vi "Eye Movement Analyser.vi"(7 "Data Output":T12) -> ()   [LabVIEW 2016] (continued)
                  w295 = T14[] [enum."Process Coils Data"] items=["--- System ---", "Panel Monitoring", "Check Save Status", "Initialize", "Initialise GUI", "Quit", "--- Import ---", "Desaccade Time Data", "Desaccade Time Data Background", "Paint Delete", "Load Batch Log File", "Make Batch List", "Update Batch List", "Delete Batch List", "Delete Temporary LVS", "Save Temporary LVS", "Check for Batch LVS", "Process 3D Chinchilla", "Find default parameter", "Mars3D old", "Chair", "EyeSeeCam", "Open last session", "Save RAW", "Auto Impulse Parameter", "Save Image", "Wireless", "Process Coils Data", "Process JHOC Data", "Process Animal Data", "Australian Data", "ASCII", "Mars 3D", "Mars 3D Training", "Position Mean Plugin", "plot generator plugin", "Human VOG system", "Optotrak", "spline", "COR", "galvanic", "Generate New Time Plot", "Make off and gains permanent", "Generate New Impulse Plot", "Defer Impulse Plot", "Fill Impulse Plot Data", "Scale Impulse Plot", "Un-Defer Impulse Plot", "Snap Impulse Cursor", "Extract Saccades", "Impulse Analyser", "NTA", "Acceleration", "Saccade Velocity", "Horizontal Align", "Vertical Align", "Delete Impulse", "Cut Before", "Cut After", "Filter Data", "Undo Last", "Redo", "Mean and STD", "Group Analyser", "Generate Report", "Phase Plots", "Gain and Phase", "Example Plugin", "Time Constant Plugin", "Export Data", "Export Time Series Data", "Append Data", "Save Data", "Load Data", "Cut in Range", "Keep in range", "Stop"] ("State Stack (out)")
                  n169 = event-data() -> ()  [unwired: 1 in, 7 out]
                }
                event "Impulse Analyser": Mouse Up {
                  w299 = T14[] [enum."Impulse Analyser", enum."Generate New Impulse Plot"] items=["--- System ---", "Panel Monitoring", "Check Save Status", "Initialize", "Initialise GUI", "Quit", "--- Import ---", "Desaccade Time Data", "Desaccade Time Data Background", "Paint Delete", "Load Batch Log File", "Make Batch List", "Update Batch List", "Delete Batch List", "Delete Temporary LVS", "Save Temporary LVS", "Check for Batch LVS", "Process 3D Chinchilla", "Find default parameter", "Mars3D old", "Chair", "EyeSeeCam", "Open last session", "Save RAW", "Auto Impulse Parameter", "Save Image", "Wireless", "Process Coils Data", "Process JHOC Data", "Process Animal Data", "Australian Data", "ASCII", "Mars 3D", "Mars 3D Training", "Position Mean Plugin", "plot generator plugin", "Human VOG system", "Optotrak", "spline", "COR", "galvanic", "Generate New Time Plot", "Make off and gains permanent", "Generate New Impulse Plot", "Defer Impulse Plot", "Fill Impulse Plot Data", "Scale Impulse Plot", "Un-Defer Impulse Plot", "Snap Impulse Cursor", "Extract Saccades", "Impulse Analyser", "NTA", "Acceleration", "Saccade Velocity", "Horizontal Align", "Vertical Align", "Delete Impulse", "Cut Before", "Cut After", "Filter Data", "Undo Last", "Redo", "Mean and STD", "Group Analyser", "Generate Report", "Phase Plots", "Gain and Phase", "Example Plugin", "Time Constant Plugin", "Export Data", "Export Time Series Data", "Append Data", "Save Data", "Load Data", "Cut in Range", "Keep in range", "Stop"] ("State Stack (out)")
                  n170 = event-data() -> ()  [unwired: 1 in, 7 out]
                  n171 = local write "Trace"(0 ("Trace")) -> ()
                }
                event "Generate New Plot": Mouse Up {
                  w302 = T14[] [enum."Generate New Time Plot"] items=["--- System ---", "Panel Monitoring", "Check Save Status", "Initialize", "Initialise GUI", "Quit", "--- Import ---", "Desaccade Time Data", "Desaccade Time Data Background", "Paint Delete", "Load Batch Log File", "Make Batch List", "Update Batch List", "Delete Batch List", "Delete Temporary LVS", "Save Temporary LVS", "Check for Batch LVS", "Process 3D Chinchilla", "Find default parameter", "Mars3D old", "Chair", "EyeSeeCam", "Open last session", "Save RAW", "Auto Impulse Parameter", "Save Image", "Wireless", "Process Coils Data", "Process JHOC Data", "Process Animal Data", "Australian Data", "ASCII", "Mars 3D", "Mars 3D Training", "Position Mean Plugin", "plot generator plugin", "Human VOG system", "Optotrak", "spline", "COR", "galvanic", "Generate New Time Plot", "Make off and gains permanent", "Generate New Impulse Plot", "Defer Impulse Plot", "Fill Impulse Plot Data", "Scale Impulse Plot", "Un-Defer Impulse Plot", "Snap Impulse Cursor", "Extract Saccades", "Impulse Analyser", "NTA", "Acceleration", "Saccade Velocity", "Horizontal Align", "Vertical Align", "Delete Impulse", "Cut Before", "Cut After", "Filter Data", "Undo Last", "Redo", "Mean and STD", "Group Analyser", "Generate Report", "Phase Plots", "Gain and Phase", "Example Plugin", "Time Constant Plugin", "Export Data", "Export Time Series Data", "Append Data", "Save Data", "Load Data", "Cut in Range", "Keep in range", "Stop"] ("State Stack (out)")
                  n172 = event-data() -> ()  [unwired: 1 in, 7 out]
                }
                event "Impulse Plane": Value Change {
                  n173 = event-data() -> ("NewVal"=w305:bool)  [unwired: 1 in, 4 out]
                  n174 = Select(t=T16."Enabled" ("Disabled"), s=w305, f=T16."Disabled and Grayed Out" ("Disabled")) -> (s? t:f=w309:T16)
                  n175 = property on="Trigger Channel (Other)" class="Ring (strict)"("DisabledEnum"=w309, "Visible"=TRUE) -> ()  [unwired: 2 in, 2 out]
                  n176 = local write "Other Trigger channel"(w305) -> ()
                  n177 = case shown="False" w305 {
                    frame False {
                      n178 = local write "Impulse Plane 2"(T9."Yaw" ("Impulse Plane")) -> ()
                    }
                    frame True {
                      n179 = local write "Impulse Plane 2"(T9."Other" ("Impulse Plane")) -> ()
                    }
                  }
                  n180 = local write "Trace"(0 ("Trace")) -> ()
                }
                event "Trace": Value Change {
                  w316 = T14[] [enum."Generate New Impulse Plot"] items=["--- System ---", "Panel Monitoring", "Check Save Status", "Initialize", "Initialise GUI", "Quit", "--- Import ---", "Desaccade Time Data", "Desaccade Time Data Background", "Paint Delete", "Load Batch Log File", "Make Batch List", "Update Batch List", "Delete Batch List", "Delete Temporary LVS", "Save Temporary LVS", "Check for Batch LVS", "Process 3D Chinchilla", "Find default parameter", "Mars3D old", "Chair", "EyeSeeCam", "Open last session", "Save RAW", "Auto Impulse Parameter", "Save Image", "Wireless", "Process Coils Data", "Process JHOC Data", "Process Animal Data", "Australian Data", "ASCII", "Mars 3D", "Mars 3D Training", "Position Mean Plugin", "plot generator plugin", "Human VOG system", "Optotrak", "spline", "COR", "galvanic", "Generate New Time Plot", "Make off and gains permanent", "Generate New Impulse Plot", "Defer Impulse Plot", "Fill Impulse Plot Data", "Scale Impulse Plot", "Un-Defer Impulse Plot", "Snap Impulse Cursor", "Extract Saccades", "Impulse Analyser", "NTA", "Acceleration", "Saccade Velocity", "Horizontal Align", "Vertical Align", "Delete Impulse", "Cut Before", "Cut After", "Filter Data", "Undo Last", "Redo", "Mean and STD", "Group Analyser", "Generate Report", "Phase Plots", "Gain and Phase", "Example Plugin", "Time Constant Plugin", "Export Data", "Export Time Series Data", "Append Data", "Save Data", "Load Data", "Cut in Range", "Keep in range", "Stop"] ("State Stack (out)")
                  n181 = event-data() -> ()  [unwired: 1 in, 5 out]
                }
                event "Analyze Saccades": Mouse Down {
                  w319 = T14[] [enum."Desaccade Time Data"] items=["--- System ---", "Panel Monitoring", "Check Save Status", "Initialize", "Initialise GUI", "Quit", "--- Import ---", "Desaccade Time Data", "Desaccade Time Data Background", "Paint Delete", "Load Batch Log File", "Make Batch List", "Update Batch List", "Delete Batch List", "Delete Temporary LVS", "Save Temporary LVS", "Check for Batch LVS", "Process 3D Chinchilla", "Find default parameter", "Mars3D old", "Chair", "EyeSeeCam", "Open last session", "Save RAW", "Auto Impulse Parameter", "Save Image", "Wireless", "Process Coils Data", "Process JHOC Data", "Process Animal Data", "Australian Data", "ASCII", "Mars 3D", "Mars 3D Training", "Position Mean Plugin", "plot generator plugin", "Human VOG system", "Optotrak", "spline", "COR", "galvanic", "Generate New Time Plot", "Make off and gains permanent", "Generate New Impulse Plot", "Defer Impulse Plot", "Fill Impulse Plot Data", "Scale Impulse Plot", "Un-Defer Impulse Plot", "Snap Impulse Cursor", "Extract Saccades", "Impulse Analyser", "NTA", "Acceleration", "Saccade Velocity", "Horizontal Align", "Vertical Align", "Delete Impulse", "Cut Before", "Cut After", "Filter Data", "Undo Last", "Redo", "Mean and STD", "Group Analyser", "Generate Report", "Phase Plots", "Gain and Phase", "Example Plugin", "Time Constant Plugin", "Export Data", "Export Time Series Data", "Append Data", "Save Data", "Load Data", "Cut in Range", "Keep in range", "Stop"] ("State Stack (out)")
                  n182 = event-data() -> ()  [unwired: 1 in, 7 out]
                }
                event "Capture Saccade": Value Change {
                  w321 = T14[] [enum."Generate New Impulse Plot"] items=["--- System ---", "Panel Monitoring", "Check Save Status", "Initialize", "Initialise GUI", "Quit", "--- Import ---", "Desaccade Time Data", "Desaccade Time Data Background", "Paint Delete", "Load Batch Log File", "Make Batch List", "Update Batch List", "Delete Batch List", "Delete Temporary LVS", "Save Temporary LVS", "Check for Batch LVS", "Process 3D Chinchilla", "Find default parameter", "Mars3D old", "Chair", "EyeSeeCam", "Open last session", "Save RAW", "Auto Impulse Parameter", "Save Image", "Wireless", "Process Coils Data", "Process JHOC Data", "Process Animal Data", "Australian Data", "ASCII", "Mars 3D", "Mars 3D Training", "Position Mean Plugin", "plot generator plugin", "Human VOG system", "Optotrak", "spline", "COR", "galvanic", "Generate New Time Plot", "Make off and gains permanent", "Generate New Impulse Plot", "Defer Impulse Plot", "Fill Impulse Plot Data", "Scale Impulse Plot", "Un-Defer Impulse Plot", "Snap Impulse Cursor", "Extract Saccades", "Impulse Analyser", "NTA", "Acceleration", "Saccade Velocity", "Horizontal Align", "Vertical Align", "Delete Impulse", "Cut Before", "Cut After", "Filter Data", "Undo Last", "Redo", "Mean and STD", "Group Analyser", "Generate Report", "Phase Plots", "Gain and Phase", "Example Plugin", "Time Constant Plugin", "Export Data", "Export Time Series Data", "Append Data", "Save Data", "Load Data", "Cut in Range", "Keep in range", "Stop"] ("State Stack (out)")
                  n183 = event-data() -> ()  [unwired: 1 in, 5 out]
                }
                event "Options", "Help": Value Change {
                  n184 = event-data() -> ()  [unwired: 1 in, 5 out]
                  n185 = local read "Options"() -> (w326:bool)
                  n186 = case shown="False" w326 {
                    tunnel: [w327 enum32{"Page 1", "Page 3", "Page 2"}."Page 2" ("Tab Control Impuls")] -> w325
                    frame False {
                      n187 = local read "Help"() -> (w328:bool)
                      n188 = case shown="True" w328 {
                        tunnel: [enum32{"Page 1", "Page 3", "Page 2"}."Page 1" ("Tab Control Impuls") enum32{"Page 1", "Page 3", "Page 2"}."Page 3" ("Tab Control Impuls")] -> w327
                        frame False {
                        }
                        frame True {
                        }
                      }
                    }
                    frame True {
                    }
                  }
                  n189 = local write "Tab Control Impuls"(w325) -> ()
                }
                event "Impulse Characteristic from Cursor": Mouse Up {
                  n190 = event-data() -> ()  [unwired: 1 in, 7 out]
                  n191 = property on="Time series Trace" class="WFGraph (strict)"("Active Cursor"=u32 1) -> ("Cursor.Cursor X"=w338:dbl, "Cursor.Cursor Y"=w345:dbl)  [unwired: 2 in, 2 out]
                  n192 = property on="Time series Trace" class="WFGraph (strict)"("Active Cursor"=u32 0) -> ("Cursor.Cursor X"=w335:dbl, "Cursor.Cursor Y"=w346:dbl)  [unwired: 2 in, 2 out]
                  n193 = Multiply(x=w338, y=1000.0) -> (x*y=w337:dbl)
                  n194 = Multiply(x=w335, y=1000.0) -> (x*y=w334:dbl)
                  n195 = property on="Impulse surround" class="Clust (strict)"() -> ("Value"=w353:T6)  [unwired: 2 in, 2 out]
                  n196 = Subtract(x=w337, y=w334) -> (x-y=w350:dbl)
                  n197 = Max & Min(x=w346, y=w345) -> (max(x,y)=w343:dbl)  [unwired: 1 out]
                  n198 = Divide(x=w350, y=2.0) -> (x/y=w358:dbl)
                  n199 = Multiply(x=w350, y=0.2) -> (x*y=w347:dbl)
                  n200 = Multiply(x=w350, y=1.2) -> (x*y=w348:dbl)
                  n201 = property on="Impulse Characteristics" class="Clust (strict)"() -> ("Value"=w355:T7)  [unwired: 2 in, 2 out]
                  n202 = Bundle By Name(cluster=w353, "Pre Impulse (ms)"=w347, "Post Impulse (ms)"=w348) -> (w352:T6)
                  n203 = Multiply(x=w343, y=0.7) -> (x*y=w341:dbl)
                  n204 = Multiply(x=w343, y=1.3) -> (x*y=w340:dbl)
                  n205 = Multiply(x=w358, y=0.8) -> (x*y=w354:dbl)
                  n206 = property on="Impulse surround" class="Clust (strict)"("Value"=w352) -> ()  [unwired: 2 in, 2 out]
                  n207 = Bundle By Name(cluster=w355, "Min Vel /Trigger"=w341, "Maximum Velocity"=w340, "Width / Offset (ms)"=w354) -> (w356:T7)
                  n208 = property on="Impulse Characteristics" class="Clust (strict)"("Value"=w356) -> ()  [unwired: 2 in, 2 out]
                }
                event "Add Autosort": Mouse Up {
                  n209 = event-data() -> ()  [unwired: 1 in, 7 out]
                  n210 = property on="Autosize Parameter Set" class="Ring (strict)"() -> ("Value"=w365:i8)  [unwired: 2 in, 2 out]
                  n211 = Equal To 0?(x=w365) -> (x = 0?=w364:bool)
                  n212 = case shown="False" w364 {
                    frame False {
                      w366 = TRUE ("Visible")
                      w367 = FALSE ("Visible")
                      w369 = TRUE ("Visible")
                      n213 = property on="Add Autosort OK" class="Bool (strict)"("Visible"=w369) -> ()  [unwired: 2 in, 2 out]
                      n214 = property on="Add Autosort Cancel" class="Bool (strict)"("Visible"=w369) -> ()  [unwired: 2 in, 2 out]
                      n215 = property on="Add Autosort" class="Bool (strict)"("Visible"=w367) -> ()  [unwired: 2 in, 2 out]
                      n216 = property on="Del Autosort" class="Bool (strict)"("Visible"=w367) -> ()  [unwired: 2 in, 2 out]
                      n217 = property on="Autosort Name" class="Str"("Visible"=w369, "Value"="" ("Autosort Name")) -> ()  [unwired: 2 in, 2 out]
                      n218 = property on="Default" class="Bool (strict)"("Visible"=w366, "Value"=w366) -> ()  [unwired: 2 in, 2 out]
                    }
                    frame True {
                      n219 = One Button Dialog(message="No Parameter-Set selected! Please select an Auto-Sort Parameter-Set by using a Load-Data Program like Mars 3D. ") -> ()  [unwired: 1 in, 1 out]
                    }
                  }
                }
                event "Add Autosort Cancel": Mouse Up {
                  w372 = FALSE ("Visible")
                  w374 = TRUE ("Visible")
                  w375 = FALSE ("Visible")
                  n220 = event-data() -> ()  [unwired: 1 in, 7 out]
                  n221 = property on="Add Autosort OK" class="Bool (strict)"("Visible"=w375) -> ()  [unwired: 2 in, 2 out]
                  n222 = property on="Add Autosort Cancel" class="Bool (strict)"("Visible"=w375) -> ()  [unwired: 2 in, 2 out]
                  n223 = property on="Add Autosort" class="Bool (strict)"("Visible"=w374) -> ()  [unwired: 2 in, 2 out]
                  n224 = property on="Autosort Name" class="Str"("Visible"=w375) -> ()  [unwired: 2 in, 2 out]
                  n225 = property on="Del Autosort" class="Bool (strict)"("Visible"=w374) -> ()  [unwired: 2 in, 2 out]
                  n226 = property on="Default" class="Bool (strict)"("Visible"=w372, "Value"=w372) -> ()  [unwired: 2 in, 2 out]
                }
                event "Add Autosort OK": Mouse Up {
                  w387 = TRUE ("Visible")
                  w388 = FALSE ("Visible")
                  n227 = event-data() -> ()  [unwired: 1 in, 7 out]
                  n228 = control-ref of="Autosize Parameter Set"() -> (w383:refnum<vi>)
                  n229 = control-ref of="Autosort Name"() -> (w381:refnum<vi>)
                  n230 = control-ref of="Cross Correlation"() -> (w376:refnum<vi>)
                  n231 = control-ref of="Impulse surround"() -> (w380:refnum<vi>)
                  n232 = control-ref of="Impulse Characteristics"() -> (w379:refnum<vi>)
                  n233 = control-ref of="Trigger Channel (Other)"() -> (w378:refnum<vi>)
                  n234 = control-ref of="Impulse Plane"() -> (w377:refnum<vi>)
                  n235 = call "Add Autosort OK pressed.vi"("Ring in"=w383, "Default"="Default", "Data OUT"=w386, "Str Refnum"=w381, "reference 5"=w376, "reference"=w380, "reference 2"=w379, "reference 3"=w378, "reference 4"=w377) -> ()  [unwired: 7 in]
                  n236 = property on="Autosort Name" class="Str"("Visible"=w388) -> ()  [unwired: 2 in, 2 out]
                  n237 = property on="Add Autosort OK" class="Bool (strict)"("Visible"=w388) -> ()  [unwired: 2 in, 2 out]
                  n238 = property on="Add Autosort Cancel" class="Bool (strict)"("Visible"=w388) -> ()  [unwired: 2 in, 2 out]
                  n239 = property on="Add Autosort" class="Bool (strict)"("Visible"=w387) -> ()  [unwired: 2 in, 2 out]
                  n240 = property on="Del Autosort" class="Bool (strict)"("Visible"=w387) -> ()  [unwired: 2 in, 2 out]
                  n241 = property on="Default" class="Bool (strict)"("Visible"=FALSE) -> ()  [unwired: 2 in, 2 out]
                }
                event "Del Autosort": Mouse Up {
                  w393 = TRUE ("Visible")
                  w394 = FALSE ("Visible")
                  n242 = event-data() -> ()  [unwired: 1 in, 7 out]
                  n243 = control-ref of="Autosize Parameter Set"() -> (w390:refnum<vi>)
                  n244 = control-ref of="Auto Sort Parameter"() -> (w389:refnum<vi>)
                  n245 = call "Autosort Delete pressed.vi"("Data OUT"=w392, "reference"=w389, "Ring in"=w390) -> ()  [unwired: 9 in]
                  n246 = property on="Autosort Name" class="Str"("Visible"=w394) -> ()  [unwired: 2 in, 2 out]
                  n247 = property on="Add Autosort OK" class="Bool (strict)"("Visible"=w394) -> ()  [unwired: 2 in, 2 out]
                  n248 = property on="Add Autosort Cancel" class="Bool (strict)"("Visible"=w394) -> ()  [unwired: 2 in, 2 out]
                  n249 = property on="Add Autosort" class="Bool (strict)"("Visible"=w393) -> ()  [unwired: 2 in, 2 out]
                  n250 = property on="Del Autosort" class="Bool (strict)"("Visible"=w393) -> ()  [unwired: 2 in, 2 out]
                }
                event "Autosize Parameter Set": Value Change {
                  n251 = event-data() -> ("NewVal"=w401:i8)  [unwired: 1 in, 4 out]
                  n252 = Not Equal?(x=w401, y=i8 0) -> (x != y?=w395:bool)
                  n253 = property on="Add Autosort" class="Bool (strict)"("Visible"=w395) -> ()  [unwired: 2 in, 2 out]
                  n254 = property on="Del Autosort" class="Bool (strict)"("Visible"=w395) -> ()  [unwired: 2 in, 2 out]
                  n255 = control-ref of="Auto Sort Parameter"() -> (w396:refnum<vi>)
                  n256 = call "Autosort Parameter Set selected.vi"("NewVal"=w401, "Data OUT"=w399, "Ring in"=w396) -> ("State stack IN"=w398:T14[])  [unwired: 8 in]
                }
                event "Filter Data": Mouse Up {
                  w403 = T14[] [enum."Filter Data", enum."Generate New Time Plot"] items=["--- System ---", "Panel Monitoring", "Check Save Status", "Initialize", "Initialise GUI", "Quit", "--- Import ---", "Desaccade Time Data", "Desaccade Time Data Background", "Paint Delete", "Load Batch Log File", "Make Batch List", "Update Batch List", "Delete Batch List", "Delete Temporary LVS", "Save Temporary LVS", "Check for Batch LVS", "Process 3D Chinchilla", "Find default parameter", "Mars3D old", "Chair", "EyeSeeCam", "Open last session", "Save RAW", "Auto Impulse Parameter", "Save Image", "Wireless", "Process Coils Data", "Process JHOC Data", "Process Animal Data", "Australian Data", "ASCII", "Mars 3D", "Mars 3D Training", "Position Mean Plugin", "plot generator plugin", "Human VOG system", "Optotrak", "spline", "COR", "galvanic", "Generate New Time Plot", "Make off and gains permanent", "Generate New Impulse Plot", "Defer Impulse Plot", "Fill Impulse Plot Data", "Scale Impulse Plot", "Un-Defer Impulse Plot", "Snap Impulse Cursor", "Extract Saccades", "Impulse Analyser", "NTA", "Acceleration", "Saccade Velocity", "Horizontal Align", "Vertical Align", "Delete Impulse", "Cut Before", "Cut After", "Filter Data", "Undo Last", "Redo", "Mean and STD", "Group Analyser", "Generate Report", "Phase Plots", "Gain and Phase", "Example Plugin", "Time Constant Plugin", "Export Data", "Export Time Series Data", "Append Data", "Save Data", "Load Data", "Cut in Range", "Keep in range", "Stop"] ("State Stack (out)")
                  n257 = event-data() -> ()  [unwired: 1 in, 7 out]
                }
                event "Generate New Impulse Plot": Mouse Up {
                  w406 = T14[] [enum."Generate New Impulse Plot"] items=["--- System ---", "Panel Monitoring", "Check Save Status", "Initialize", "Initialise GUI", "Quit", "--- Import ---", "Desaccade Time Data", "Desaccade Time Data Background", "Paint Delete", "Load Batch Log File", "Make Batch List", "Update Batch List", "Delete Batch List", "Delete Temporary LVS", "Save Temporary LVS", "Check for Batch LVS", "Process 3D Chinchilla", "Find default parameter", "Mars3D old", "Chair", "EyeSeeCam", "Open last session", "Save RAW", "Auto Impulse Parameter", "Save Image", "Wireless", "Process Coils Data", "Process JHOC Data", "Process Animal Data", "Australian Data", "ASCII", "Mars 3D", "Mars 3D Training", "Position Mean Plugin", "plot generator plugin", "Human VOG system", "Optotrak", "spline", "COR", "galvanic", "Generate New Time Plot", "Make off and gains permanent", "Generate New Impulse Plot", "Defer Impulse Plot", "Fill Impulse Plot Data", "Scale Impulse Plot", "Un-Defer Impulse Plot", "Snap Impulse Cursor", "Extract Saccades", "Impulse Analyser", "NTA", "Acceleration", "Saccade Velocity", "Horizontal Align", "Vertical Align", "Delete Impulse", "Cut Before", "Cut After", "Filter Data", "Undo Last", "Redo", "Mean and STD", "Group Analyser", "Generate Report", "Phase Plots", "Gain and Phase", "Example Plugin", "Time Constant Plugin", "Export Data", "Export Time Series Data", "Append Data", "Save Data", "Load Data", "Cut in Range", "Keep in range", "Stop"] ("State Stack (out)")
                  n258 = event-data() -> ()  [unwired: 1 in, 7 out]
                }
                event "Horizontal Align": Mouse Up {
                  w409 = T14[] [enum."Horizontal Align", enum."Generate New Impulse Plot"] items=["--- System ---", "Panel Monitoring", "Check Save Status", "Initialize", "Initialise GUI", "Quit", "--- Import ---", "Desaccade Time Data", "Desaccade Time Data Background", "Paint Delete", "Load Batch Log File", "Make Batch List", "Update Batch List", "Delete Batch List", "Delete Temporary LVS", "Save Temporary LVS", "Check for Batch LVS", "Process 3D Chinchilla", "Find default parameter", "Mars3D old", "Chair", "EyeSeeCam", "Open last session", "Save RAW", "Auto Impulse Parameter", "Save Image", "Wireless", "Process Coils Data", "Process JHOC Data", "Process Animal Data", "Australian Data", "ASCII", "Mars 3D", "Mars 3D Training", "Position Mean Plugin", "plot generator plugin", "Human VOG system", "Optotrak", "spline", "COR", "galvanic", "Generate New Time Plot", "Make off and gains permanent", "Generate New Impulse Plot", "Defer Impulse Plot", "Fill Impulse Plot Data", "Scale Impulse Plot", "Un-Defer Impulse Plot", "Snap Impulse Cursor", "Extract Saccades", "Impulse Analyser", "NTA", "Acceleration", "Saccade Velocity", "Horizontal Align", "Vertical Align", "Delete Impulse", "Cut Before", "Cut After", "Filter Data", "Undo Last", "Redo", "Mean and STD", "Group Analyser", "Generate Report", "Phase Plots", "Gain and Phase", "Example Plugin", "Time Constant Plugin", "Export Data", "Export Time Series Data", "Append Data", "Save Data", "Load Data", "Cut in Range", "Keep in range", "Stop"] ("State Stack (out)")
                  n259 = event-data() -> ()  [unwired: 1 in, 7 out]
                }
                event "Vertical Align": Mouse Up {
                  w412 = T14[] [enum."Vertical Align", enum."Generate New Impulse Plot"] items=["--- System ---", "Panel Monitoring", "Check Save Status", "Initialize", "Initialise GUI", "Quit", "--- Import ---", "Desaccade Time Data", "Desaccade Time Data Background", "Paint Delete", "Load Batch Log File", "Make Batch List", "Update Batch List", "Delete Batch List", "Delete Temporary LVS", "Save Temporary LVS", "Check for Batch LVS", "Process 3D Chinchilla", "Find default parameter", "Mars3D old", "Chair", "EyeSeeCam", "Open last session", "Save RAW", "Auto Impulse Parameter", "Save Image", "Wireless", "Process Coils Data", "Process JHOC Data", "Process Animal Data", "Australian Data", "ASCII", "Mars 3D", "Mars 3D Training", "Position Mean Plugin", "plot generator plugin", "Human VOG system", "Optotrak", "spline", "COR", "galvanic", "Generate New Time Plot", "Make off and gains permanent", "Generate New Impulse Plot", "Defer Impulse Plot", "Fill Impulse Plot Data", "Scale Impulse Plot", "Un-Defer Impulse Plot", "Snap Impulse Cursor", "Extract Saccades", "Impulse Analyser", "NTA", "Acceleration", "Saccade Velocity", "Horizontal Align", "Vertical Align", "Delete Impulse", "Cut Before", "Cut After", "Filter Data", "Undo Last", "Redo", "Mean and STD", "Group Analyser", "Generate Report", "Phase Plots", "Gain and Phase", "Example Plugin", "Time Constant Plugin", "Export Data", "Export Time Series Data", "Append Data", "Save Data", "Load Data", "Cut in Range", "Keep in range", "Stop"] ("State Stack (out)")
                  n260 = event-data() -> ()  [unwired: 1 in, 7 out]
                }
                event "Delete Impulse": Mouse Up {
                  w415 = T14[] [enum."Delete Impulse", enum."Generate New Impulse Plot"] items=["--- System ---", "Panel Monitoring", "Check Save Status", "Initialize", "Initialise GUI", "Quit", "--- Import ---", "Desaccade Time Data", "Desaccade Time Data Background", "Paint Delete", "Load Batch Log File", "Make Batch List", "Update Batch List", "Delete Batch List", "Delete Temporary LVS", "Save Temporary LVS", "Check for Batch LVS", "Process 3D Chinchilla", "Find default parameter", "Mars3D old", "Chair", "EyeSeeCam", "Open last session", "Save RAW", "Auto Impulse Parameter", "Save Image", "Wireless", "Process Coils Data", "Process JHOC Data", "Process Animal Data", "Australian Data", "ASCII", "Mars 3D", "Mars 3D Training", "Position Mean Plugin", "plot generator plugin", "Human VOG system", "Optotrak", "spline", "COR", "galvanic", "Generate New Time Plot", "Make off and gains permanent", "Generate New Impulse Plot", "Defer Impulse Plot", "Fill Impulse Plot Data", "Scale Impulse Plot", "Un-Defer Impulse Plot", "Snap Impulse Cursor", "Extract Saccades", "Impulse Analyser", "NTA", "Acceleration", "Saccade Velocity", "Horizontal Align", "Vertical Align", "Delete Impulse", "Cut Before", "Cut After", "Filter Data", "Undo Last", "Redo", "Mean and STD", "Group Analyser", "Generate Report", "Phase Plots", "Gain and Phase", "Example Plugin", "Time Constant Plugin", "Export Data", "Export Time Series Data", "Append Data", "Save Data", "Load Data", "Cut in Range", "Keep in range", "Stop"] ("State Stack (out)")
                  n261 = event-data() -> ()  [unwired: 1 in, 7 out]
                }
                event Key Down {
                  n262 = event-data() -> ("Char"=w422:i16, "VKey"=w426:T33, "PlatMods"=w417:T34)  [unwired: 1 in, 6 out]
                  n263 = Type Cast(type="", x=w422) -> (*(type *) &x=w420:string)
                  n264 = String Subset(string=w420, offset (0)=1) -> (substring=w418:string)  [unwired: 1 in]
                  n265 = case shown="\"Delete\", \"Escape\"" w426 {
                    tunnel: [w429 w435 w441 w443 _] -> w424
                    tunnel: w418 -> [w428 _ _ _ _]
                    tunnel: w417 -> [w427 _ _ _ _]
                    frame "ASCII", Default {
                      n266 = case shown="\"g\"" w428 {
                        tunnel: [w430 w433] -> w429
                        tunnel: w427 -> [_ w432]
                        frame "", Default {
                          w430 = T14[] [enum."Panel Monitoring"] items=["--- System ---", "Panel Monitoring", "Check Save Status", "Initialize", "Initialise GUI", "Quit", "--- Import ---", "Desaccade Time Data", "Desaccade Time Data Background", "Paint Delete", "Load Batch Log File", "Make Batch List", "Update Batch List", "Delete Batch List", "Delete Temporary LVS", "Save Temporary LVS", "Check for Batch LVS", "Process 3D Chinchilla", "Find default parameter", "Mars3D old", "Chair", "EyeSeeCam", "Open last session", "Save RAW", "Auto Impulse Parameter", "Save Image", "Wireless", "Process Coils Data", "Process JHOC Data", "Process Animal Data", "Australian Data", "ASCII", "Mars 3D", "Mars 3D Training", "Position Mean Plugin", "plot generator plugin", "Human VOG system", "Optotrak", "spline", "COR", "galvanic", "Generate New Time Plot", "Make off and gains permanent", "Generate New Impulse Plot", "Defer Impulse Plot", "Fill Impulse Plot Data", "Scale Impulse Plot", "Un-Defer Impulse Plot", "Snap Impulse Cursor", "Extract Saccades", "Impulse Analyser", "NTA", "Acceleration", "Saccade Velocity", "Horizontal Align", "Vertical Align", "Delete Impulse", "Cut Before", "Cut After", "Filter Data", "Undo Last", "Redo", "Mean and STD", "Group Analyser", "Generate Report", "Phase Plots", "Gain and Phase", "Example Plugin", "Time Constant Plugin", "Export Data", "Export Time Series Data", "Append Data", "Save Data", "Load Data", "Cut in Range", "Keep in range", "Stop"] ("State Stack (out)")
                        }
                        frame "g" {
                          n267 = Unbundle By Name(w432) -> ("Ctrl"=w431:bool)
                          n268 = case shown="True" w431 {
                            tunnel: [_ w434] -> w433
                            frame False {
                            }
                            frame True {
                              w434 = T14[] [enum."Gain and Phase"] items=["--- System ---", "Panel Monitoring", "Check Save Status", "Initialize", "Initialise GUI", "Quit", "--- Import ---", "Desaccade Time Data", "Desaccade Time Data Background", "Paint Delete", "Load Batch Log File", "Make Batch List", "Update Batch List", "Delete Batch List", "Delete Temporary LVS", "Save Temporary LVS", "Check for Batch LVS", "Process 3D Chinchilla", "Find default parameter", "Mars3D old", "Chair", "EyeSeeCam", "Open last session", "Save RAW", "Auto Impulse Parameter", "Save Image", "Wireless", "Process Coils Data", "Process JHOC Data", "Process Animal Data", "Australian Data", "ASCII", "Mars 3D", "Mars 3D Training", "Position Mean Plugin", "plot generator plugin", "Human VOG system", "Optotrak", "spline", "COR", "galvanic", "Generate New Time Plot", "Make off and gains permanent", "Generate New Impulse Plot", "Defer Impulse Plot", "Fill Impulse Plot Data", "Scale Impulse Plot", "Un-Defer Impulse Plot", "Snap Impulse Cursor", "Extract Saccades", "Impulse Analyser", "NTA", "Acceleration", "Saccade Velocity", "Horizontal Align", "Vertical Align", "Delete Impulse", "Cut Before", "Cut After", "Filter Data", "Undo Last", "Redo", "Mean and STD", "Group Analyser", "Generate Report", "Phase Plots", "Gain and Phase", "Example Plugin", "Time Constant Plugin", "Export Data", "Export Time Series Data", "Append Data", "Save Data", "Load Data", "Cut in Range", "Keep in range", "Stop"] ("State Stack (out)")
                            }
                          }
                        }
                      }
                    }
                    frame "Up" {
                      w435 = T14[] [enum."Generate New Impulse Plot"] items=["--- System ---", "Panel Monitoring", "Check Save Status", "Initialize", "Initialise GUI", "Quit", "--- Import ---", "Desaccade Time Data", "Desaccade Time Data Background", "Paint Delete", "Load Batch Log File", "Make Batch List", "Update Batch List", "Delete Batch List", "Delete Temporary LVS", "Save Temporary LVS", "Check for Batch LVS", "Process 3D Chinchilla", "Find default parameter", "Mars3D old", "Chair", "EyeSeeCam", "Open last session", "Save RAW", "Auto Impulse Parameter", "Save Image", "Wireless", "Process Coils Data", "Process JHOC Data", "Process Animal Data", "Australian Data", "ASCII", "Mars 3D", "Mars 3D Training", "Position Mean Plugin", "plot generator plugin", "Human VOG system", "Optotrak", "spline", "COR", "galvanic", "Generate New Time Plot", "Make off and gains permanent", "Generate New Impulse Plot", "Defer Impulse Plot", "Fill Impulse Plot Data", "Scale Impulse Plot", "Un-Defer Impulse Plot", "Snap Impulse Cursor", "Extract Saccades", "Impulse Analyser", "NTA", "Acceleration", "Saccade Velocity", "Horizontal Align", "Vertical Align", "Delete Impulse", "Cut Before", "Cut After", "Filter Data", "Undo Last", "Redo", "Mean and STD", "Group Analyser", "Generate Report", "Phase Plots", "Gain and Phase", "Example Plugin", "Time Constant Plugin", "Export Data", "Export Time Series Data", "Append Data", "Save Data", "Load Data", "Cut in Range", "Keep in range", "Stop"] ("State Stack (out)")
                      n269 = local read "Trace"() -> (w437:i32)
                      n270 = Increment(x=w437) -> (x+1=w436:i32)
                      n271 = local write "Trace"(w436) -> ()
                    }
                    frame "Down" {
                      w441 = T14[] [enum."Generate New Impulse Plot"] items=["--- System ---", "Panel Monitoring", "Check Save Status", "Initialize", "Initialise GUI", "Quit", "--- Import ---", "Desaccade Time Data", "Desaccade Time Data Background", "Paint Delete", "Load Batch Log File", "Make Batch List", "Update Batch List", "Delete Batch List", "Delete Temporary LVS", "Save Temporary LVS", "Check for Batch LVS", "Process 3D Chinchilla", "Find default parameter", "Mars3D old", "Chair", "EyeSeeCam", "Open last session", "Save RAW", "Auto Impulse Parameter", "Save Image", "Wireless", "Process Coils Data", "Process JHOC Data", "Process Animal Data", "Australian Data", "ASCII", "Mars 3D", "Mars 3D Training", "Position Mean Plugin", "plot generator plugin", "Human VOG system", "Optotrak", "spline", "COR", "galvanic", "Generate New Time Plot", "Make off and gains permanent", "Generate New Impulse Plot", "Defer Impulse Plot", "Fill Impulse Plot Data", "Scale Impulse Plot", "Un-Defer Impulse Plot", "Snap Impulse Cursor", "Extract Saccades", "Impulse Analyser", "NTA", "Acceleration", "Saccade Velocity", "Horizontal Align", "Vertical Align", "Delete Impulse", "Cut Before", "Cut After", "Filter Data", "Undo Last", "Redo", "Mean and STD", "Group Analyser", "Generate Report", "Phase Plots", "Gain and Phase", "Example Plugin", "Time Constant Plugin", "Export Data", "Export Time Series Data", "Append Data", "Save Data", "Load Data", "Cut in Range", "Keep in range", "Stop"] ("State Stack (out)")
                      n272 = local read "Trace"() -> (w442:i32)
                      n273 = Decrement(x=w442) -> (x-1=w440:i32)
                      n274 = Max & Min(x=w440, y=0) -> (max(x,y)=w438:i32)  [unwired: 1 out]
                      n275 = local write "Trace"(w438) -> ()
                    }
                    frame "Delete", "Escape" {
                      w443 = T14[] [enum."Delete Impulse", enum."Generate New Impulse Plot", enum."Panel Monitoring"] items=["--- System ---", "Panel Monitoring", "Check Save Status", "Initialize", "Initialise GUI", "Quit", "--- Import ---", "Desaccade Time Data", "Desaccade Time Data Background", "Paint Delete", "Load Batch Log File", "Make Batch List", "Update Batch List", "Delete Batch List", "Delete Temporary LVS", "Save Temporary LVS", "Check for Batch LVS", "Process 3D Chinchilla", "Find default parameter", "Mars3D old", "Chair", "EyeSeeCam", "Open last session", "Save RAW", "Auto Impulse Parameter", "Save Image", "Wireless", "Process Coils Data", "Process JHOC Data", "Process Animal Data", "Australian Data", "ASCII", "Mars 3D", "Mars 3D Training", "Position Mean Plugin", "plot generator plugin", "Human VOG system", "Optotrak", "spline", "COR", "galvanic", "Generate New Time Plot", "Make off and gains permanent", "Generate New Impulse Plot", "Defer Impulse Plot", "Fill Impulse Plot Data", "Scale Impulse Plot", "Un-Defer Impulse Plot", "Snap Impulse Cursor", "Extract Saccades", "Impulse Analyser", "NTA", "Acceleration", "Saccade Velocity", "Horizontal Align", "Vertical Align", "Delete Impulse", "Cut Before", "Cut After", "Filter Data", "Undo Last", "Redo", "Mean and STD", "Group Analyser", "Generate Report", "Phase Plots", "Gain and Phase", "Example Plugin", "Time Constant Plugin", "Export Data", "Export Time Series Data", "Append Data", "Save Data", "Load Data", "Cut in Range", "Keep in range", "Stop"] ("State Stack (out)")
                    }
                    frame "F9" {
                      n276 = local read "Mean and STD"() -> (w445:bool)
                      n277 = Not(x=w445) -> (.not. x?=w444:bool)
                      n278 = property on="Mean and STD" class="Bool (strict)"("Val(Sgnl)"=w444) -> ()  [unwired: 2 in, 2 out]
                    }
                  }
                }
                event "Impulse Trace": Mouse Wheel {
                  w457 = 1.1  # Zoom Speed
                  # "Select zoom type"
                  # "Mouse Wheel Zoom"
                  # "Zoom algorithm maintains the ratio between the mouse location and the bottom left corner of the plot."
                  # "Negative delta zooms out\ni.e. Zoom between 0 - 1"
                  n279 = event-data() -> ("CtlRef"=w478:refnum<vi>, "Coords"=w477:T27, "Delta"=w458:i32, "PlatMods"=w453:T34)  [unwired: 1 in, 1 out]
                  n280 = Unbundle By Name(w453) -> ("Alt"=w452:bool, "Ctrl"=w449:bool)
                  n281 = invoke class="WFGraph (strict)" method="Map Coords To XY"(reference=w478, "Coords"=w477) -> (reference out=w476:refnum<vi>, error out=w475:errorcluster, "XY"=w470:cluster{"X":dbl, "Y":dbl})  [unwired: 5 in, 4 out]
                  n282 = Negate(x=w458) -> (-x=w454:i32)
                  n283 = Multiply(x=w454, y=w457) -> (x*y=w456:dbl)
                  n284 = Select(t=enum16{"Both", "Horizontal", "Vertical"}."Vertical", s=w452, f=enum16{"Both", "Horizontal", "Vertical"}."Both") -> (s? t:f=w447:enum16{"Both", "Horizontal", "Vertical"})
                  n285 = Negate(x=w456) -> (-x=w460:dbl)
                  n286 = property class="WFGraph (strict)"(reference=w476, error in=w475) -> (reference out=w466:refnum<vi>, error out=w467:errorcluster, "XScale.Maximum"=w474:dbl, "XScale.Minimum"=w473:dbl, "YScale.Maximum"=w472:dbl, "YScale.Minimum"=w471:dbl)
                  n287 = Unbundle By Name(w470) -> ("X"=w469:dbl, "Y"=w468:dbl)
                  n288 = Reciprocal(x=w460) -> (1/x=w459:dbl)
                  n289 = Greater Or Equal To 0?(x=w456) -> (x >= 0?=w461:bool)
                  n290 = Select(t=enum16{"Both", "Horizontal", "Vertical"}."Horizontal", s=w449, f=w447) -> (s? t:f=w446:enum16{"Both", "Horizontal", "Vertical"})
                  n291 = Select(t=w456, s=w461, f=w459) -> (s? t:f=w455:dbl)
                  n292 = formula code="W0 = Xmax0-Xmin0;\nW1 = W0*Zoom;\nXmin1 = x + (W1/W0)*(Xmin0 - x);\nXmax1 = Xmin1 + W1;\n\n\nH0 = Ymax0-Ymin0;\nH1 = H0*Zoom;\nYmin1 = y + (H1/H0)*(Ymin0 - y);\nYmax1 = Ymin1 + H1;"("Xmax0"=w474, "Xmin0"=w473, "Ymax0"=w472, "Ymin0"=w471, "x"=w469, "y"=w468, "Zoom"=w455) -> ("Xmin1"=w464:dbl, "Xmax1"=w465:dbl, "Ymax1"=w463:dbl, "Ymin1"=w462:dbl)  [unwired: 4 out]
                  n293 = case shown="\"Vertical\"" w446 {
                    tunnel: w467 -> [w486 w490 w494]
                    tunnel: w466 -> [w485 w489 w493]
                    tunnel: w465 -> [w484 w488 _]
                    tunnel: w464 -> [w483 w487 _]
                    tunnel: w463 -> [w482 _ w492]
                    tunnel: w462 -> [w481 _ w491]
                    frame "Both", Default {
                      n294 = property class="WFGraph (strict)"(reference=w485, error in=w486, "XScale.Maximum"=w484, "XScale.Minimum"=w483, "YScale.Maximum"=w482, "YScale.Minimum"=w481) -> ()  [unwired: 2 out]
                    }
                    frame "Horizontal" {
                      n295 = property class="WFGraph (strict)"(reference=w489, error in=w490, "XScale.Maximum"=w488, "XScale.Minimum"=w487) -> ()  [unwired: 2 out]
                    }
                    frame "Vertical" {
                      n296 = property class="WFGraph (strict)"(reference=w493, error in=w494, "YScale.Maximum"=w492, "YScale.Minimum"=w491) -> ()  [unwired: 2 out]
                    }
                  }
                }
                event "Undo Last": Mouse Up {
                  w496 = T14[] [enum."Undo Last", enum."Generate New Impulse Plot"] items=["--- System ---", "Panel Monitoring", "Check Save Status", "Initialize", "Initialise GUI", "Quit", "--- Import ---", "Desaccade Time Data", "Desaccade Time Data Background", "Paint Delete", "Load Batch Log File", "Make Batch List", "Update Batch List", "Delete Batch List", "Delete Temporary LVS", "Save Temporary LVS", "Check for Batch LVS", "Process 3D Chinchilla", "Find default parameter", "Mars3D old", "Chair", "EyeSeeCam", "Open last session", "Save RAW", "Auto Impulse Parameter", "Save Image", "Wireless", "Process Coils Data", "Process JHOC Data", "Process Animal Data", "Australian Data", "ASCII", "Mars 3D", "Mars 3D Training", "Position Mean Plugin", "plot generator plugin", "Human VOG system", "Optotrak", "spline", "COR", "galvanic", "Generate New Time Plot", "Make off and gains permanent", "Generate New Impulse Plot", "Defer Impulse Plot", "Fill Impulse Plot Data", "Scale Impulse Plot", "Un-Defer Impulse Plot", "Snap Impulse Cursor", "Extract Saccades", "Impulse Analyser", "NTA", "Acceleration", "Saccade Velocity", "Horizontal Align", "Vertical Align", "Delete Impulse", "Cut Before", "Cut After", "Filter Data", "Undo Last", "Redo", "Mean and STD", "Group Analyser", "Generate Report", "Phase Plots", "Gain and Phase", "Example Plugin", "Time Constant Plugin", "Export Data", "Export Time Series Data", "Append Data", "Save Data", "Load Data", "Cut in Range", "Keep in range", "Stop"] ("State Stack (out)")
                  n297 = event-data() -> ()  [unwired: 1 in, 7 out]
                }
                event "Redo": Mouse Up {
                  w499 = T14[] [enum."Redo", enum."Generate New Impulse Plot"] items=["--- System ---", "Panel Monitoring", "Check Save Status", "Initialize", "Initialise GUI", "Quit", "--- Import ---", "Desaccade Time Data", "Desaccade Time Data Background", "Paint Delete", "Load Batch Log File", "Make Batch List", "Update Batch List", "Delete Batch List", "Delete Temporary LVS", "Save Temporary LVS", "Check for Batch LVS", "Process 3D Chinchilla", "Find default parameter", "Mars3D old", "Chair", "EyeSeeCam", "Open last session", "Save RAW", "Auto Impulse Parameter", "Save Image", "Wireless", "Process Coils Data", "Process JHOC Data", "Process Animal Data", "Australian Data", "ASCII", "Mars 3D", "Mars 3D Training", "Position Mean Plugin", "plot generator plugin", "Human VOG system", "Optotrak", "spline", "COR", "galvanic", "Generate New Time Plot", "Make off and gains permanent", "Generate New Impulse Plot", "Defer Impulse Plot", "Fill Impulse Plot Data", "Scale Impulse Plot", "Un-Defer Impulse Plot", "Snap Impulse Cursor", "Extract Saccades", "Impulse Analyser", "NTA", "Acceleration", "Saccade Velocity", "Horizontal Align", "Vertical Align", "Delete Impulse", "Cut Before", "Cut After", "Filter Data", "Undo Last", "Redo", "Mean and STD", "Group Analyser", "Generate Report", "Phase Plots", "Gain and Phase", "Example Plugin", "Time Constant Plugin", "Export Data", "Export Time Series Data", "Append Data", "Save Data", "Load Data", "Cut in Range", "Keep in range", "Stop"] ("State Stack (out)")
                  n298 = event-data() -> ()  [unwired: 1 in, 7 out]
                }
                event "Cut Before": Mouse Up {
                  w502 = T14[] [enum."Cut Before", enum."Generate New Impulse Plot"] items=["--- System ---", "Panel Monitoring", "Check Save Status", "Initialize", "Initialise GUI", "Quit", "--- Import ---", "Desaccade Time Data", "Desaccade Time Data Background", "Paint Delete", "Load Batch Log File", "Make Batch List", "Update Batch List", "Delete Batch List", "Delete Temporary LVS", "Save Temporary LVS", "Check for Batch LVS", "Process 3D Chinchilla", "Find default parameter", "Mars3D old", "Chair", "EyeSeeCam", "Open last session", "Save RAW", "Auto Impulse Parameter", "Save Image", "Wireless", "Process Coils Data", "Process JHOC Data", "Process Animal Data", "Australian Data", "ASCII", "Mars 3D", "Mars 3D Training", "Position Mean Plugin", "plot generator plugin", "Human VOG system", "Optotrak", "spline", "COR", "galvanic", "Generate New Time Plot", "Make off and gains permanent", "Generate New Impulse Plot", "Defer Impulse Plot", "Fill Impulse Plot Data", "Scale Impulse Plot", "Un-Defer Impulse Plot", "Snap Impulse Cursor", "Extract Saccades", "Impulse Analyser", "NTA", "Acceleration", "Saccade Velocity", "Horizontal Align", "Vertical Align", "Delete Impulse", "Cut Before", "Cut After", "Filter Data", "Undo Last", "Redo", "Mean and STD", "Group Analyser", "Generate Report", "Phase Plots", "Gain and Phase", "Example Plugin", "Time Constant Plugin", "Export Data", "Export Time Series Data", "Append Data", "Save Data", "Load Data", "Cut in Range", "Keep in range", "Stop"] ("State Stack (out)")
                  n299 = event-data() -> ()  [unwired: 1 in, 7 out]
                }
                event "Cut After": Mouse Up {
                  w505 = T14[] [enum."Cut After", enum."Generate New Impulse Plot"] items=["--- System ---", "Panel Monitoring", "Check Save Status", "Initialize", "Initialise GUI", "Quit", "--- Import ---", "Desaccade Time Data", "Desaccade Time Data Background", "Paint Delete", "Load Batch Log File", "Make Batch List", "Update Batch List", "Delete Batch List", "Delete Temporary LVS", "Save Temporary LVS", "Check for Batch LVS", "Process 3D Chinchilla", "Find default parameter", "Mars3D old", "Chair", "EyeSeeCam", "Open last session", "Save RAW", "Auto Impulse Parameter", "Save Image", "Wireless", "Process Coils Data", "Process JHOC Data", "Process Animal Data", "Australian Data", "ASCII", "Mars 3D", "Mars 3D Training", "Position Mean Plugin", "plot generator plugin", "Human VOG system", "Optotrak", "spline", "COR", "galvanic", "Generate New Time Plot", "Make off and gains permanent", "Generate New Impulse Plot", "Defer Impulse Plot", "Fill Impulse Plot Data", "Scale Impulse Plot", "Un-Defer Impulse Plot", "Snap Impulse Cursor", "Extract Saccades", "Impulse Analyser", "NTA", "Acceleration", "Saccade Velocity", "Horizontal Align", "Vertical Align", "Delete Impulse", "Cut Before", "Cut After", "Filter Data", "Undo Last", "Redo", "Mean and STD", "Group Analyser", "Generate Report", "Phase Plots", "Gain and Phase", "Example Plugin", "Time Constant Plugin", "Export Data", "Export Time Series Data", "Append Data", "Save Data", "Load Data", "Cut in Range", "Keep in range", "Stop"] ("State Stack (out)")
                  n300 = event-data() -> ()  [unwired: 1 in, 7 out]
                }
                event "Mean and STD": Value Change {
                  w509 = T14[] [enum."Generate New Impulse Plot"] items=["--- System ---", "Panel Monitoring", "Check Save Status", "Initialize", "Initialise GUI", "Quit", "--- Import ---", "Desaccade Time Data", "Desaccade Time Data Background", "Paint Delete", "Load Batch Log File", "Make Batch List", "Update Batch List", "Delete Batch List", "Delete Temporary LVS", "Save Temporary LVS", "Check for Batch LVS", "Process 3D Chinchilla", "Find default parameter", "Mars3D old", "Chair", "EyeSeeCam", "Open last session", "Save RAW", "Auto Impulse Parameter", "Save Image", "Wireless", "Process Coils Data", "Process JHOC Data", "Process Animal Data", "Australian Data", "ASCII", "Mars 3D", "Mars 3D Training", "Position Mean Plugin", "plot generator plugin", "Human VOG system", "Optotrak", "spline", "COR", "galvanic", "Generate New Time Plot", "Make off and gains permanent", "Generate New Impulse Plot", "Defer Impulse Plot", "Fill Impulse Plot Data", "Scale Impulse Plot", "Un-Defer Impulse Plot", "Snap Impulse Cursor", "Extract Saccades", "Impulse Analyser", "NTA", "Acceleration", "Saccade Velocity", "Horizontal Align", "Vertical Align", "Delete Impulse", "Cut Before", "Cut After", "Filter Data", "Undo Last", "Redo", "Mean and STD", "Group Analyser", "Generate Report", "Phase Plots", "Gain and Phase", "Example Plugin", "Time Constant Plugin", "Export Data", "Export Time Series Data", "Append Data", "Save Data", "Load Data", "Cut in Range", "Keep in range", "Stop"] ("State Stack (out)")
                  n301 = event-data() -> ()  [unwired: 1 in, 6 out]
                }
                event "Shortcut 1": Mouse Down {
                  w510 = T14[] [enum."Generate New Impulse Plot"] items=["--- System ---", "Panel Monitoring", "Check Save Status", "Initialize", "Initialise GUI", "Quit", "--- Import ---", "Desaccade Time Data", "Desaccade Time Data Background", "Paint Delete", "Load Batch Log File", "Make Batch List", "Update Batch List", "Delete Batch List", "Delete Temporary LVS", "Save Temporary LVS", "Check for Batch LVS", "Process 3D Chinchilla", "Find default parameter", "Mars3D old", "Chair", "EyeSeeCam", "Open last session", "Save RAW", "Auto Impulse Parameter", "Save Image", "Wireless", "Process Coils Data", "Process JHOC Data", "Process Animal Data", "Australian Data", "ASCII", "Mars 3D", "Mars 3D Training", "Position Mean Plugin", "plot generator plugin", "Human VOG system", "Optotrak", "spline", "COR", "galvanic", "Generate New Time Plot", "Make off and gains permanent", "Generate New Impulse Plot", "Defer Impulse Plot", "Fill Impulse Plot Data", "Scale Impulse Plot", "Un-Defer Impulse Plot", "Snap Impulse Cursor", "Extract Saccades", "Impulse Analyser", "NTA", "Acceleration", "Saccade Velocity", "Horizontal Align", "Vertical Align", "Delete Impulse", "Cut Before", "Cut After", "Filter Data", "Undo Last", "Redo", "Mean and STD", "Group Analyser", "Generate Report", "Phase Plots", "Gain and Phase", "Example Plugin", "Time Constant Plugin", "Export Data", "Export Time Series Data", "Append Data", "Save Data", "Load Data", "Cut in Range", "Keep in range", "Stop"] ("State Stack (out)")
                  n302 = event-data() -> ()  [unwired: 1 in, 7 out]
                  n303 = Bundle By Name(cluster=w513, "Parameter Impuls Series"=T8 [{"Color"=4652800, "Visible"=TRUE, "Channel"=1, "Invert"=FALSE, "Desaccade"=FALSE, "Offset"=0.0, "Gain"=1.0}, {"Color"=9073151, "Visible"=TRUE, "Channel"=5, "Invert"=FALSE, "Desaccade"=FALSE, "Offset"=0.0, "Gain"=1.0}, {"Color"=55791, "Visible"=TRUE, "Channel"=6, "Invert"=FALSE, "Desaccade"=FALSE, "Offset"=0.0, "Gain"=1.0}, {"Color"=16747144, "Visible"=TRUE, "Channel"=16, "Invert"=FALSE, "Desaccade"=FALSE, "Offset"=0.0, "Gain"=1.0}, {"Color"=16745794, "Visible"=TRUE, "Channel"=17, "Invert"=FALSE, "Desaccade"=FALSE, "Offset"=0.0, "Gain"=1.0}]) -> (w512:T30)
                }
                event "Shortcut 2": Mouse Down {
                  w515 = T14[] [enum."Generate New Impulse Plot"] items=["--- System ---", "Panel Monitoring", "Check Save Status", "Initialize", "Initialise GUI", "Quit", "--- Import ---", "Desaccade Time Data", "Desaccade Time Data Background", "Paint Delete", "Load Batch Log File", "Make Batch List", "Update Batch List", "Delete Batch List", "Delete Temporary LVS", "Save Temporary LVS", "Check for Batch LVS", "Process 3D Chinchilla", "Find default parameter", "Mars3D old", "Chair", "EyeSeeCam", "Open last session", "Save RAW", "Auto Impulse Parameter", "Save Image", "Wireless", "Process Coils Data", "Process JHOC Data", "Process Animal Data", "Australian Data", "ASCII", "Mars 3D", "Mars 3D Training", "Position Mean Plugin", "plot generator plugin", "Human VOG system", "Optotrak", "spline", "COR", "galvanic", "Generate New Time Plot", "Make off and gains permanent", "Generate New Impulse Plot", "Defer Impulse Plot", "Fill Impulse Plot Data", "Scale Impulse Plot", "Un-Defer Impulse Plot", "Snap Impulse Cursor", "Extract Saccades", "Impulse Analyser", "NTA", "Acceleration", "Saccade Velocity", "Horizontal Align", "Vertical Align", "Delete Impulse", "Cut Before", "Cut After", "Filter Data", "Undo Last", "Redo", "Mean and STD", "Group Analyser", "Generate Report", "Phase Plots", "Gain and Phase", "Example Plugin", "Time Constant Plugin", "Export Data", "Export Time Series Data", "Append Data", "Save Data", "Load Data", "Cut in Range", "Keep in range", "Stop"] ("State Stack (out)")
                  n304 = event-data() -> ()  [unwired: 1 in, 7 out]
                  n305 = Bundle By Name(cluster=w518, "Parameter Impuls Series"=T8 [{"Color"=4652800, "Visible"=TRUE, "Channel"=1, "Invert"=FALSE, "Desaccade"=FALSE, "Offset"=0.0, "Gain"=1.0}, {"Color"=7455743, "Visible"=TRUE, "Channel"=7, "Invert"=FALSE, "Desaccade"=FALSE, "Offset"=0.0, "Gain"=1.0}, {"Color"=7455743, "Visible"=TRUE, "Channel"=18, "Invert"=FALSE, "Desaccade"=FALSE, "Offset"=0.0, "Gain"=1.0}]) -> (w517:T30)
                }
                event "Shortcut 3": Mouse Down {
